vi "Return to Single Pulse.vi"(8 "error in (no error)":errorcluster, 11 "Main_UI in":refnum<class "Main_UI.lvclass">) -> (0 "error out":errorcluster, 3 "Main_UI out":refnum<class "Main_UI.lvclass">)   [LabVIEW 2020, in "Main_UI.lvlib" / "Main_UI.lvclass"]
uses:
  Main_UI.lvclass
  Main_UI.lvclass/Main_UI.ctl
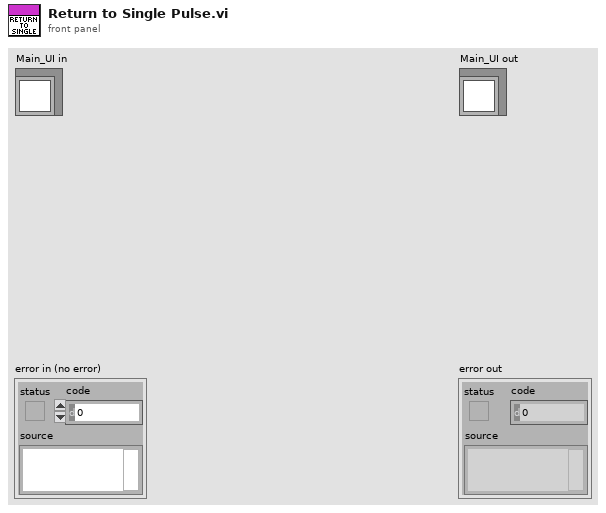
[diagram p1: front panel]
types:
  T1 = enum32{"Select Single Test", "Select Life cycle test"}
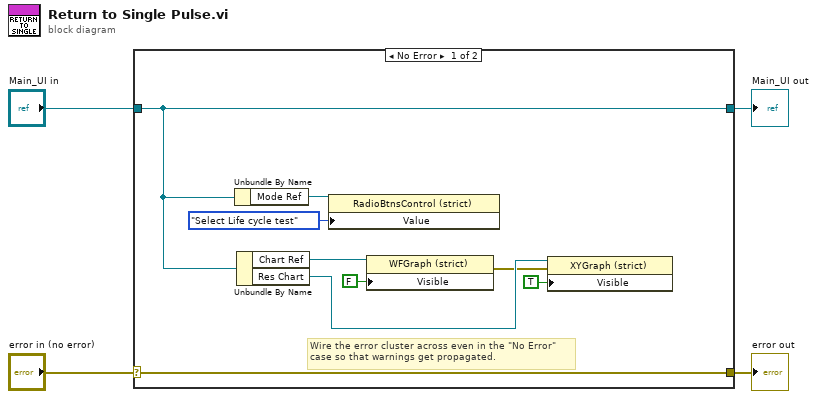
[diagram p0: block diagram]
diagram:
  n1 = case shown="No Error" "error in (no error)" {
    selector: "error in (no error)" -> [w13 w15]
    tunnel: [w13 w15] -> w3
    tunnel: [w10 w14] -> w1
    tunnel: "Main_UI in" -> [w10 w14]
    frame No Error {
      # "Wire the error cluster across even in the \"No Error\"\ncase so that warnings get propagated."
      n2 = Unbundle By Name(w10) -> ("Mode Ref"=w12:refnum<vi>)
      n3 = Unbundle By Name(w10) -> ("Chart Ref"=w9:refnum<vi>, "Res Chart"=w8:refnum<vi>)
      n4 = property class="RadioBtnsControl (strict)"(reference=w12, "Value"=T1."Select Life cycle test") -> ()  [unwired: 1 in, 2 out]
      n5 = property class="WFGraph (strict)"(reference=w9, "Visible"=FALSE) -> (error out=w7:errorcluster)  [unwired: 1 in, 1 out]
      n6 = property class="XYGraph (strict)"(reference=w8, error in=w7, "Visible"=TRUE) -> ()  [unwired: 2 out]
    }
    frame Error {
    }
  }
  "error out" <- w3
  "Main_UI out" <- w1
